vi "LockinVsgGraphs.vi"(0 "Array in":dbl[](array[numeric]), 1 "Boolean":bool, 2 "Numeric":dbl) -> (14 "Array out":cluster{"Y":dbl[], "Y":dbl[]}[](array[cluster]), 15 "Array 3":cluster{"Y":dbl[], "Y":dbl[]}[](array[cluster]))   [LabVIEW 2016, in "Transport.lvclass"]
uses:
  Transport.lvclass
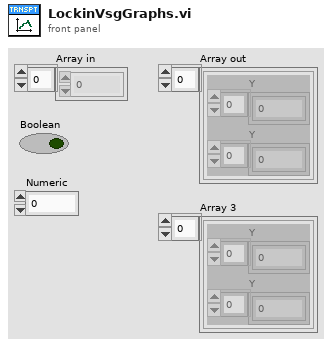
[diagram p1: front panel]
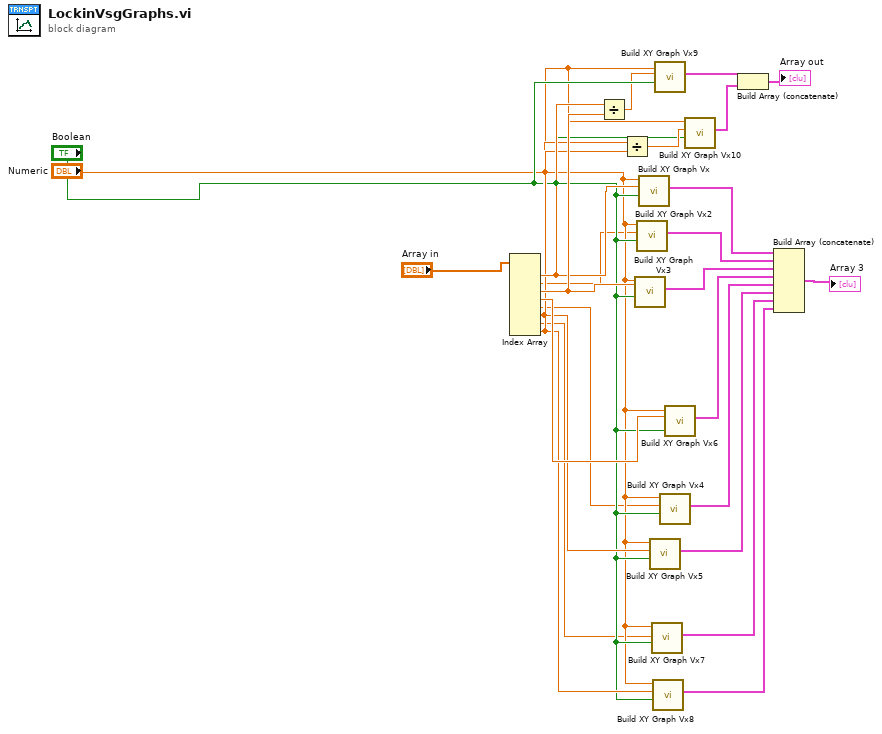
[diagram p0: block diagram]
diagram:
  n1 = Index Array(array="Array in") -> (element #1=w19:dbl, element #2=w3:dbl, element #3=w21:dbl, element #4=w20:dbl, element #5=w4:dbl, element #6=w13:dbl, element #7=w8:dbl, element #8=w14:dbl)  [unwired: 8 in]
  n2 = Divide(x=w19, y=w21) -> (x/y=w10:dbl)
  n3 = Divide(x=w13, y=w14) -> (x/y=w15:dbl)
  n4 = call "Build XY Graph Vx3"("Reset"="Boolean", "Y Input"=w21, "X Input"="Numeric") -> ("XY Graph"=w24:cluster{"Y":dbl[], "Y":dbl[]}[])  [unwired: 2 in, 6 out]
  n5 = call "Build XY Graph Vx2"("Reset"="Boolean", "Y Input"=w3, "X Input"="Numeric") -> ("XY Graph"=w2:cluster{"Y":dbl[], "Y":dbl[]}[])  [unwired: 2 in, 6 out]
  n6 = call "Build XY Graph Vx"("Reset"="Boolean", "Y Input"=w19, "X Input"="Numeric") -> ("XY Graph"=w1:cluster{"Y":dbl[], "Y":dbl[]}[])  [unwired: 2 in, 6 out]
  n7 = call "Build XY Graph Vx5"("Reset"="Boolean", "Y Input"=w13, "X Input"="Numeric") -> ("XY Graph"=w5:cluster{"Y":dbl[], "Y":dbl[]}[])  [unwired: 2 in, 6 out]
  n8 = call "Build XY Graph Vx7"("Reset"="Boolean", "Y Input"=w8, "X Input"="Numeric") -> ("XY Graph"=w6:cluster{"Y":dbl[], "Y":dbl[]}[])  [unwired: 2 in, 6 out]
  n9 = call "Build XY Graph Vx8"("Reset"="Boolean", "Y Input"=w14, "X Input"="Numeric") -> ("XY Graph"=w7:cluster{"Y":dbl[], "Y":dbl[]}[])  [unwired: 2 in, 6 out]
  n10 = call "Build XY Graph Vx9"("Reset"="Boolean", "Y Input"=w10, "X Input"="Numeric") -> ("XY Graph"=w16:cluster{"Y":dbl[], "Y":dbl[]}[])  [unwired: 2 in, 6 out]
  n11 = call "Build XY Graph Vx4"("Reset"="Boolean", "Y Input"=w4, "X Input"="Numeric") -> ("XY Graph"=w25:cluster{"Y":dbl[], "Y":dbl[]}[])  [unwired: 2 in, 6 out]
  n12 = call "Build XY Graph Vx6"("Reset"="Boolean", "Y Input"=w20, "X Input"="Numeric") -> ("XY Graph"=w23:cluster{"Y":dbl[], "Y":dbl[]}[])  [unwired: 2 in, 6 out]
  n13 = call "Build XY Graph Vx10"("Reset"="Boolean", "Y Input"=w15, "X Input"="Numeric") -> ("XY Graph"=w17:cluster{"Y":dbl[], "Y":dbl[]}[])  [unwired: 2 in, 6 out]
  n14 = Build Array (concatenate)(w16, w17) -> (→"Array out":cluster{"Y":dbl[], "Y":dbl[]}[])
  n15 = Build Array (concatenate)(w1, w2, w24, w23, w25, w5, w6, w7) -> (→"Array 3":cluster{"Y":dbl[], "Y":dbl[]}[])
